vi "Event Notification.Init Status Indicator.vi"(8 "error in (no error)":errorcluster, 10 "StatusTxtBoxRef":refnum<vi>, 11 "Event Notification in":refnum<class "Event Notification.lvclass">) -> (0 "error out":errorcluster, 3 "Event Notification out":refnum<class "Event Notification.lvclass">)   [LabVIEW 2024, in "EQMF.lvlib" / "Event Log.lvlib" / "Event Notification.lvclass"]
uses:
  Event Notification.lvclass
  Event Notification.lvclass/Event Notification.ctl
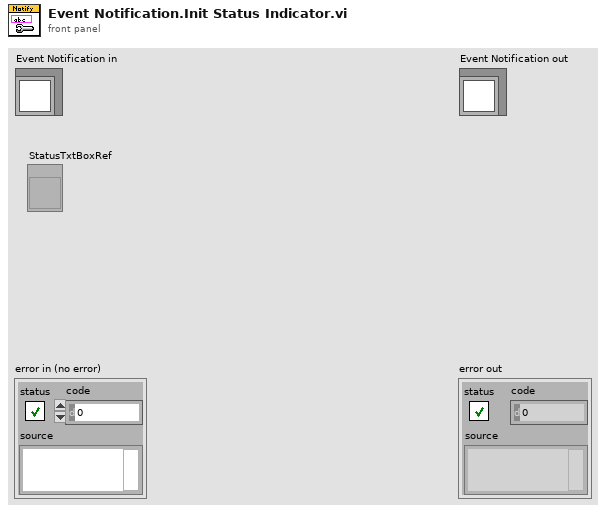
[diagram p1: front panel]
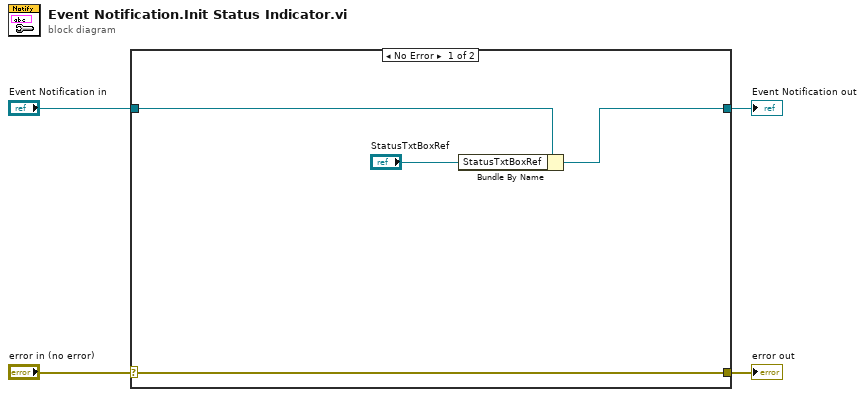
[diagram p0: block diagram]
diagram:
  n1 = case shown="No Error" "error in (no error)" {
    selector: "error in (no error)" -> [w8 w10]
    tunnel: [w8 w10] -> w3
    tunnel: [w6 w9] -> w1
    tunnel: "Event Notification in" -> [w7 w9]
    frame No Error {
      n2 = Bundle By Name(cluster=w7, "StatusTxtBoxRef"="StatusTxtBoxRef") -> (w6:refnum<class "Event Notification.lvclass">)
    }
    frame Error {
    }
  }
  "error out" <- w3
  "Event Notification out" <- w1
